vi "Traffic LightPorneet.vi"() -> ()   [LabVIEW 2013]
uses:
  SM Solution/Traffic Light/USB Template (LV 8.6)/Traffic Light/Controls/Traffic light.ctl
  SM Solution/Traffic Light/USB Template (LV 8.6)/Traffic Light/Controls/Traffic_light_left.ctl
  Controls/TLC states.ctl
panel:
  in  "North  Sensor":bool
  in  "Start":bool caption="stop"
  out "South Bound Left":T1
  out "South Bound":T2={"R"=TRUE, "Y"=FALSE, "G"=FALSE}
  out "West Bound Left":T1
  out "West Bound":T2={"R"=TRUE, "Y"=FALSE, "G"=FALSE}
  out "East Bound Left":T1
  out "East Bound":T2={"R"=TRUE, "Y"=FALSE, "G"=FALSE}
  in  "stop":bool
  in  "West Sensor":bool
  in  "East Sensor":bool
  in  "South Sensor":bool
  out "North Bound Left":T1
  out "North Bound":T2={"R"=TRUE, "Y"=FALSE, "G"=FALSE}
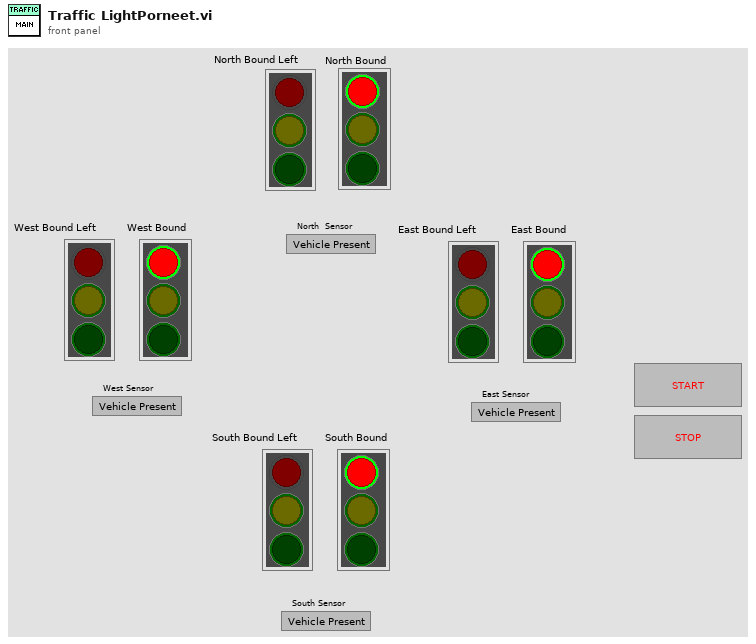
[diagram p1: front panel]
types:
  T1 = typedef "Traffic_light_left.ctl" = cluster{"R":bool, "Y":bool, "G":bool}
  T2 = typedef "Traffic light.ctl" = cluster{"R":bool, "Y":bool, "G":bool}
  T3 = cluster{"East Bound":T2, "West Bound":T2, "North Bound":T2, "South Bound":T2, "East Bound Left":T1, "West Bound Left":T1, "North Bound Left":T1, "South Bound Left":T1}
  T4 = typedef "TLC states.ctl" = enum16{"Initialize", "Start", "NS Green", "NS Yellow", "EW Green", "EW Yellow", "NS Left Green", "NS Left Yellow", "EW Left Green", "EW Left Yellow", "Stop"}
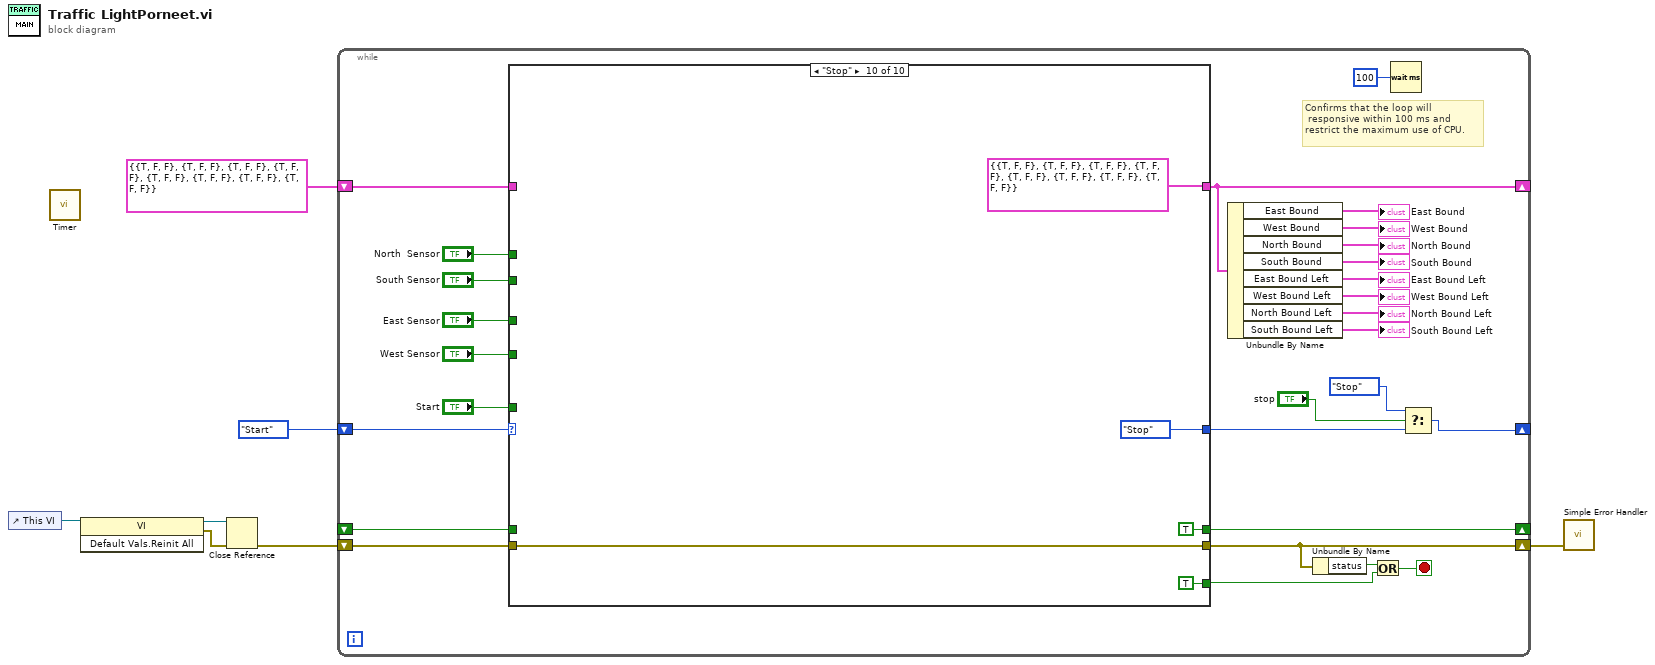
[diagram p0: block diagram]
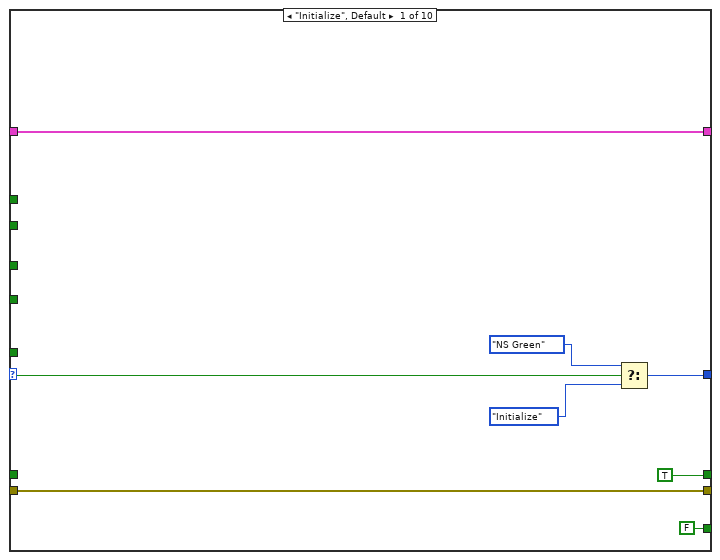
[diagram p2: hidden frame]
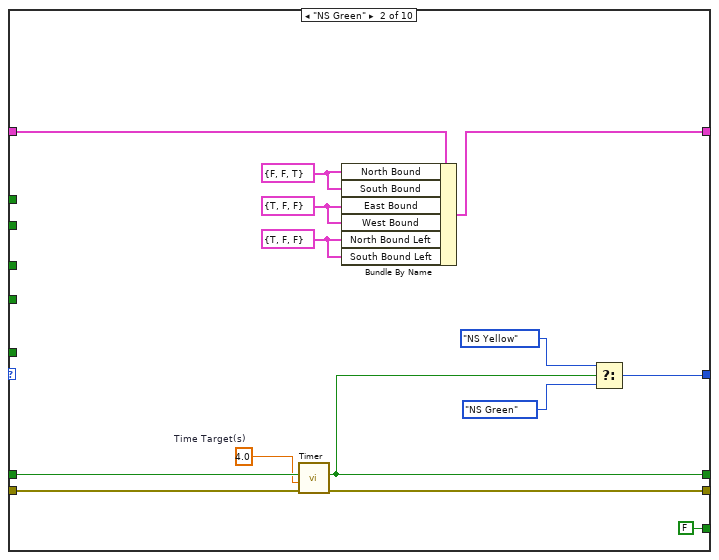
[diagram p3: hidden frame]
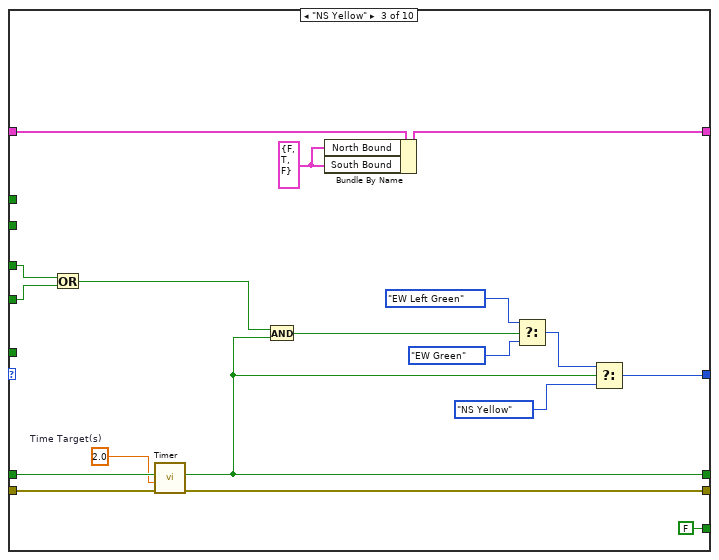
[diagram p4: hidden frame]
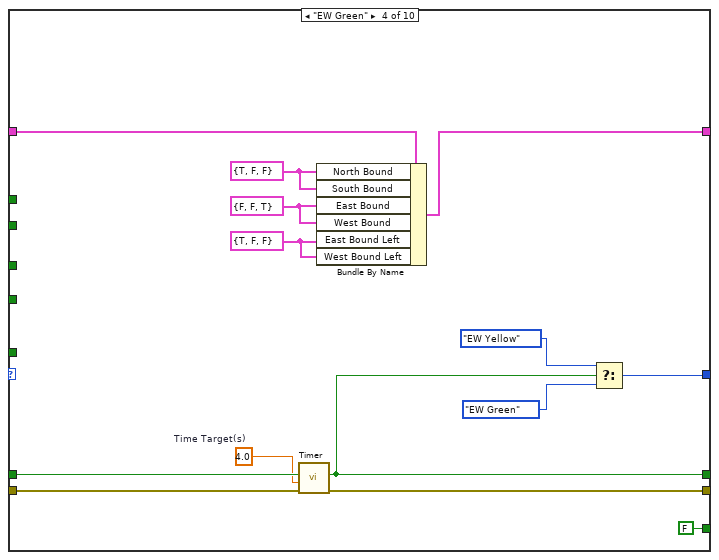
[diagram p5: hidden frame]
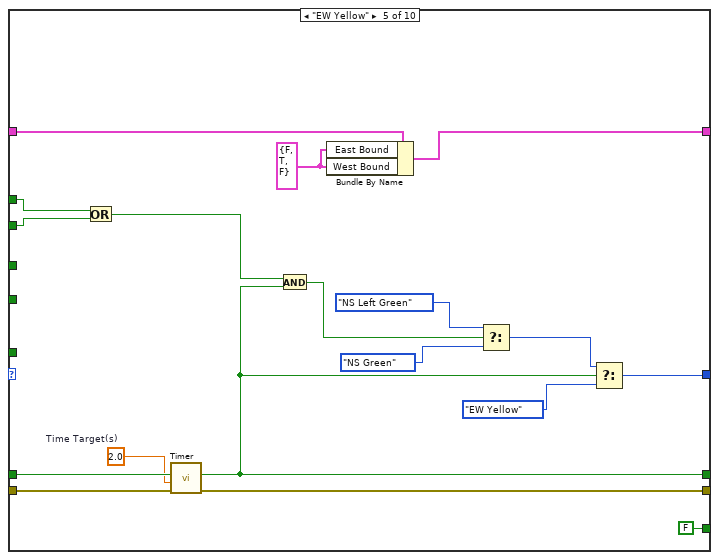
[diagram p6: hidden frame]
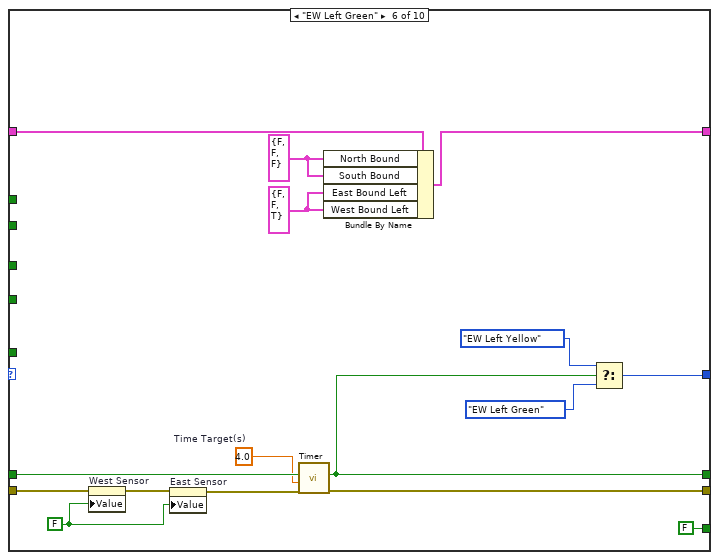
[diagram p7: hidden frame]
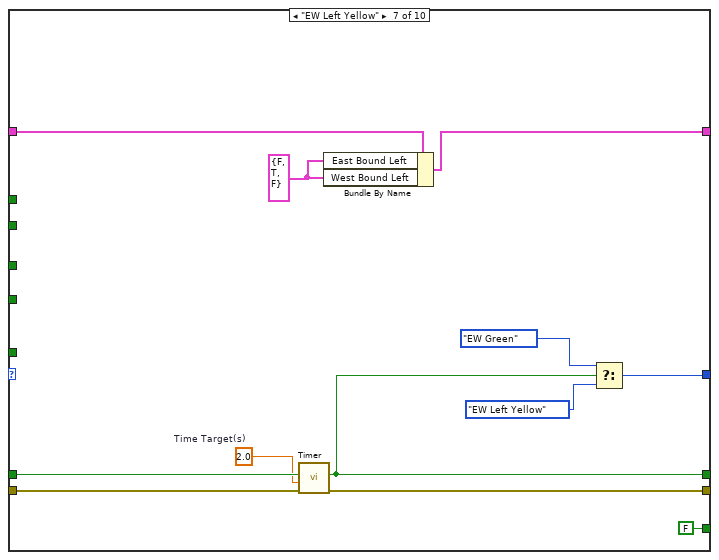
[diagram p8: hidden frame]
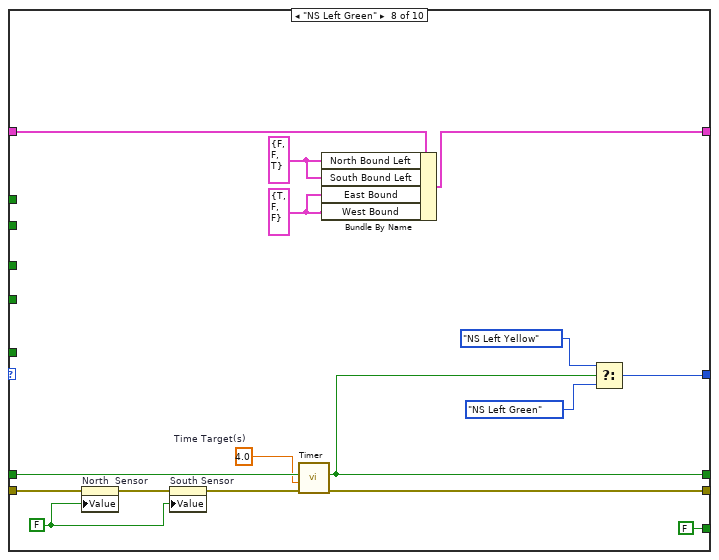
[diagram p9: hidden frame]
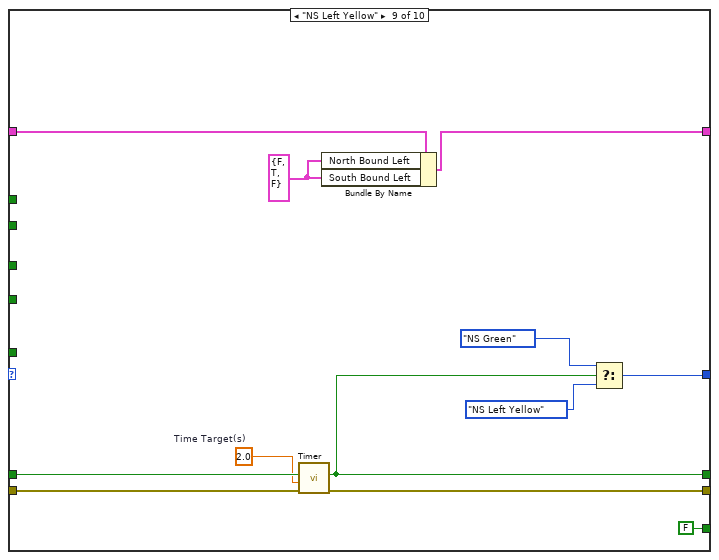
[diagram p10: hidden frame]
diagram:
  n1 = control-ref of="This VI"() -> (w7:refnum<vi>)
  n2 = call "Timer.vi"() -> ()  [unwired: 9 in, 3 out]
  n3 = invoke class="VI" method="Default Vals.Reinit All"(reference=w7) -> (reference out=w6:refnum<vi>, error out=w5:errorcluster)  [unwired: 2 in, 1 out]
  n4 = Close Reference(reference=w6, error in (no error)=w5) -> (error out=w3:errorcluster)
  n5 = while {
    shift-right: [w34] -> w4
    shift-left: w3 -> [w30]
    shift-right: [w25] -> _
    shift-left: _ -> [w24]
    shift-right: [w14] -> _
    shift-left: TLC_states."Start" ("States") -> [w29]
    shift-right: [w23] -> _
    shift-left: T3 {"East Bound"={"R"=TRUE, "Y"=FALSE, "G"=FALSE}, "West Bound"={"R"=TRUE, "Y"=FALSE, "G"=FALSE}, "North Bound"={"R"=TRUE, "Y"=FALSE, "G"=FALSE}, "South Bound"={"R"=TRUE, "Y"=FALSE, "G"=FALSE}, "East Bound Left"={"R"=TRUE, "Y"=FALSE, "G"=FALSE}, "West Bound Left"={"R"=TRUE, "Y"=FALSE, "G"=FALSE}, "North Bound Left"={"R"=TRUE, "Y"=FALSE, "G"=FALSE}, "South Bound Left"={"R"=TRUE, "Y"=FALSE, "G"=FALSE}} -> [w27]
    stop <- w33 stop-if-true
    # "Confirms that the loop will\n responsive within 100 ms and\nrestrict the maximum use of CPU."
    n6 = case shown="\"Stop\"" w29 {
      tunnel: [w42 w54 w72 w86 w104 w121 w132 w149 w160 w168] -> w34
      tunnel: [FALSE ("stop") FALSE ("stop") FALSE ("stop") FALSE ("stop") FALSE ("stop") FALSE ("stop") FALSE ("stop") FALSE ("stop") FALSE ("stop") TRUE ("stop")] -> w31
      tunnel: w30 -> [w42 w55 w73 w87 w105 w110 w133 w138 w161 w168]
      tunnel: [w37 w51 w69 w83 w101 w118 w129 w146 w157 TLC_states."Stop" ("States")] -> w28
      tunnel: [w41 w47 w67 w79 w99 w114 w125 w142 w153 T3 {"East Bound"={"R"=TRUE, "Y"=FALSE, "G"=FALSE}, "West Bound"={"R"=TRUE, "Y"=FALSE, "G"=FALSE}, "North Bound"={"R"=TRUE, "Y"=FALSE, "G"=FALSE}, "South Bound"={"R"=TRUE, "Y"=FALSE, "G"=FALSE}, "East Bound Left"={"R"=TRUE, "Y"=FALSE, "G"=FALSE}, "West Bound Left"={"R"=TRUE, "Y"=FALSE, "G"=FALSE}, "North Bound Left"={"R"=TRUE, "Y"=FALSE, "G"=FALSE}, "South Bound Left"={"R"=TRUE, "Y"=FALSE, "G"=FALSE}}] -> w23
      tunnel: w27 -> [w41 w56 w74 w88 w106 w122 w134 w150 w162 _]
      tunnel: "Start" -> [w40 _ _ _ _ _ _ _ _ _]
      tunnel: [TRUE w48 w62 w80 w94 w115 w126 w143 w154 TRUE ("Elapsed?")] -> w25
      tunnel: w24 -> [_ w53 w71 w85 w103 w120 w131 w148 w159 _]
      tunnel: "East Sensor" -> [_ _ w65 _ _ _ _ _ _ _]
      tunnel: "West Sensor" -> [_ _ w64 _ _ _ _ _ _ _]
      tunnel: "North  Sensor" -> [_ _ _ _ w97 _ _ _ _ _]
      tunnel: "South Sensor" -> [_ _ _ _ w96 _ _ _ _ _]
      frame "Initialize", Default {
        n7 = Select(t=TLC_states."NS Green" ("States"), s=w40, f=TLC_states."Initialize" ("States")) -> (s? t:f=w37:T4)
      }
      frame "NS Green" {
        w44 = T1 {"R"=TRUE, "Y"=FALSE, "G"=FALSE} ("South Bound Left")
        w45 = T2 {"R"=TRUE, "Y"=FALSE, "G"=FALSE} ("East Bound")
        w46 = T2 {"R"=FALSE, "Y"=FALSE, "G"=TRUE} ("North Bound")
        w52 = 4.0  # Time Target(s)
        n8 = call "Timer.vi"("error in (no error)"=w55, "Time Target(s)"=w52, "Reset"=w53) -> ("error out"=w54:errorcluster, "Elapsed?"=w48:bool)  [unwired: 6 in, 1 out]
        n9 = Bundle By Name(cluster=w56, "North Bound"=w46, "South Bound"=w46, "East Bound"=w45, "West Bound"=w45, "North Bound Left"=w44, "South Bound Left"=w44) -> (w47:T3)
        n10 = Select(t=TLC_states."NS Yellow" ("States"), s=w48, f=TLC_states."NS Green" ("States")) -> (s? t:f=w51:T4)
      }
      frame "NS Yellow" {
        w66 = T2 {"R"=FALSE, "Y"=TRUE, "G"=FALSE} ("North Bound")
        w70 = 2.0  # Time Target(s)
        n11 = Or(x=w65, y=w64) -> (x .or. y?=w63:bool)
        n12 = call "Timer.vi"("error in (no error)"=w73, "Time Target(s)"=w70, "Reset"=w71) -> ("error out"=w72:errorcluster, "Elapsed?"=w62:bool)  [unwired: 6 in, 1 out]
        n13 = And(x=w63, y=w62) -> (x .and. y?=w61:bool)
        n14 = Bundle By Name(cluster=w74, "North Bound"=w66, "South Bound"=w66) -> (w67:T3)
        n15 = Select(t=TLC_states."EW Left Green", s=w61, f=TLC_states."EW Green" ("States")) -> (s? t:f=w58:T4)
        n16 = Select(t=w58, s=w62, f=TLC_states."NS Yellow" ("States")) -> (s? t:f=w69:T4)
      }
      frame "EW Green" {
        w76 = T1 {"R"=TRUE, "Y"=FALSE, "G"=FALSE} ("East Bound Left")
        w77 = T2 {"R"=FALSE, "Y"=FALSE, "G"=TRUE} ("East Bound")
        w78 = T2 {"R"=TRUE, "Y"=FALSE, "G"=FALSE} ("North Bound")
        w84 = 4.0  # Time Target(s)
        n17 = call "Timer.vi"("error in (no error)"=w87, "Time Target(s)"=w84, "Reset"=w85) -> ("error out"=w86:errorcluster, "Elapsed?"=w80:bool)  [unwired: 6 in, 1 out]
        n18 = Bundle By Name(cluster=w88, "North Bound"=w78, "South Bound"=w78, "East Bound"=w77, "West Bound"=w77, "East Bound Left"=w76, "West Bound Left"=w76) -> (w79:T3)
        n19 = Select(t=TLC_states."EW Yellow" ("States"), s=w80, f=TLC_states."EW Green" ("States")) -> (s? t:f=w83:T4)
      }
      frame "EW Yellow" {
        w98 = T2 {"R"=FALSE, "Y"=TRUE, "G"=FALSE} ("East Bound")
        w102 = 2.0  # Time Target(s)
        n20 = Or(x=w97, y=w96) -> (x .or. y?=w95:bool)
        n21 = call "Timer.vi"("error in (no error)"=w105, "Time Target(s)"=w102, "Reset"=w103) -> ("error out"=w104:errorcluster, "Elapsed?"=w94:bool)  [unwired: 6 in, 1 out]
        n22 = And(x=w95, y=w94) -> (x .and. y?=w93:bool)
        n23 = Bundle By Name(cluster=w106, "East Bound"=w98, "West Bound"=w98) -> (w99:T3)
        n24 = Select(t=TLC_states."NS Left Green" ("States"), s=w93, f=TLC_states."NS Green" ("States")) -> (s? t:f=w90:T4)
        n25 = Select(t=w90, s=w94, f=TLC_states."EW Yellow" ("States")) -> (s? t:f=w101:T4)
      }
      frame "EW Left Green" {
        w108 = FALSE
        w112 = T1 {"R"=FALSE, "Y"=FALSE, "G"=TRUE} ("East Bound Left")
        w113 = T2 {"R"=FALSE, "Y"=FALSE, "G"=FALSE} ("East Bound")
        w119 = 4.0  # Time Target(s)
        n26 = property on="West Sensor" class="Bool (strict)"(error in=w110, "Value"=w108) -> (error out=w111:errorcluster)  [unwired: 1 in, 1 out]
        n27 = property on="East Sensor" class="Bool (strict)"(error in=w111, "Value"=w108) -> (error out=w109:errorcluster)  [unwired: 1 in, 1 out]
        n28 = call "Timer.vi"("error in (no error)"=w109, "Time Target(s)"=w119, "Reset"=w120) -> ("error out"=w121:errorcluster, "Elapsed?"=w115:bool)  [unwired: 6 in, 1 out]
        n29 = Bundle By Name(cluster=w122, "North Bound"=w113, "South Bound"=w113, "East Bound Left"=w112, "West Bound Left"=w112) -> (w114:T3)
        n30 = Select(t=TLC_states."EW Left Yellow" ("States"), s=w115, f=TLC_states."EW Left Green" ("States")) -> (s? t:f=w118:T4)
      }
      frame "EW Left Yellow" {
        w124 = T1 {"R"=FALSE, "Y"=TRUE, "G"=FALSE} ("East Bound Left")
        w130 = 2.0  # Time Target(s)
        n31 = call "Timer.vi"("error in (no error)"=w133, "Time Target(s)"=w130, "Reset"=w131) -> ("error out"=w132:errorcluster, "Elapsed?"=w126:bool)  [unwired: 6 in, 1 out]
        n32 = Bundle By Name(cluster=w134, "East Bound Left"=w124, "West Bound Left"=w124) -> (w125:T3)
        n33 = Select(t=TLC_states."EW Green" ("States"), s=w126, f=TLC_states."EW Left Yellow" ("States")) -> (s? t:f=w129:T4)
      }
      frame "NS Left Green" {
        w136 = FALSE
        w140 = T2 {"R"=TRUE, "Y"=FALSE, "G"=FALSE} ("East Bound")
        w141 = T1 {"R"=FALSE, "Y"=FALSE, "G"=TRUE} ("East Bound Left")
        w147 = 4.0  # Time Target(s)
        n34 = property on="North  Sensor" class="Bool (strict)"(error in=w138, "Value"=w136) -> (error out=w139:errorcluster)  [unwired: 1 in, 1 out]
        n35 = property on="South Sensor" class="Bool (strict)"(error in=w139, "Value"=w136) -> (error out=w137:errorcluster)  [unwired: 1 in, 1 out]
        n36 = call "Timer.vi"("error in (no error)"=w137, "Time Target(s)"=w147, "Reset"=w148) -> ("error out"=w149:errorcluster, "Elapsed?"=w143:bool)  [unwired: 6 in, 1 out]
        n37 = Bundle By Name(cluster=w150, "North Bound Left"=w141, "South Bound Left"=w141, "East Bound"=w140, "West Bound"=w140) -> (w142:T3)
        n38 = Select(t=TLC_states."NS Left Yellow" ("States"), s=w143, f=TLC_states."NS Left Green" ("States")) -> (s? t:f=w146:T4)
      }
      frame "NS Left Yellow" {
        w152 = T1 {"R"=FALSE, "Y"=TRUE, "G"=FALSE} ("East Bound Left")
        w158 = 2.0  # Time Target(s)
        n39 = call "Timer.vi"("error in (no error)"=w161, "Time Target(s)"=w158, "Reset"=w159) -> ("error out"=w160:errorcluster, "Elapsed?"=w154:bool)  [unwired: 6 in, 1 out]
        n40 = Bundle By Name(cluster=w162, "North Bound Left"=w152, "South Bound Left"=w152) -> (w153:T3)
        n41 = Select(t=TLC_states."NS Green" ("States"), s=w154, f=TLC_states."NS Left Yellow" ("States")) -> (s? t:f=w157:T4)
      }
      frame "Stop" {
      }
    }
    n42 = Unbundle By Name(w23) -> ("East Bound"=→"East Bound":T2, "West Bound"=→"West Bound":T2, "North Bound"=→"North Bound":T2, "South Bound"=→"South Bound":T2, "East Bound Left"=→"East Bound Left":T1, "West Bound Left"=→"West Bound Left":T1, "North Bound Left"=→"North Bound Left":T1, "South Bound Left"=→"South Bound Left":T1)
    n43 = Unbundle By Name(w34) -> ("status"=w32:bool)
    n44 = Or(x=w32, y=w31) -> (x .or. y?=w33:bool)
    n45 = Wait (ms)(milliseconds to wait=u32 100) -> ()  [unwired: 1 out]
    n46 = Select(t=TLC_states."Stop", s="stop", f=w28) -> (s? t:f=w14:T4)
  }
  n47 = call <vilib>:"Simple Error Handler.vi"("error in (no error)"=w4) -> ()  [unwired: 4 in, 5 out]
